vi "get wavefront.vi"(8 "error in":errorcluster, 11 "HasoSlopes in":refnum<class "HasoSlopes.lvclass">) -> (0 "error out":errorcluster, 1 "Pupil (new)":refnum<class "Pupil.lvclass">, 2 "Phase":refnum<class "Phase.lvclass">, 3 "HasoData out":refnum<class "HasoData.lvclass">, 5 "ComputePhaseSet.lvclass 2":refnum<class "ComputePhaseSet.lvclass">)   [LabVIEW 2020]
uses:
  Pupil.lvclass
  Phase.lvclass
  HasoSlopes.lvclass
  ComputePhaseSet.lvclass
  HasoData.lvclass
  WavefrontReconstructionMode.ctl
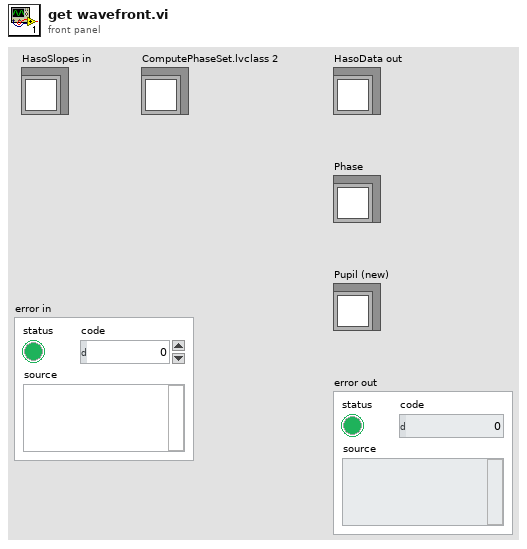
[diagram p1: front panel]
types:
  T1 = typedef "WavefrontReconstructionMode.ctl" = enum16{"None", "Modal_Legendre", "Modal_Zernike", "Zonal", "Modal_Zonal_Zernike", "Modal_Zonal_Legendre"}
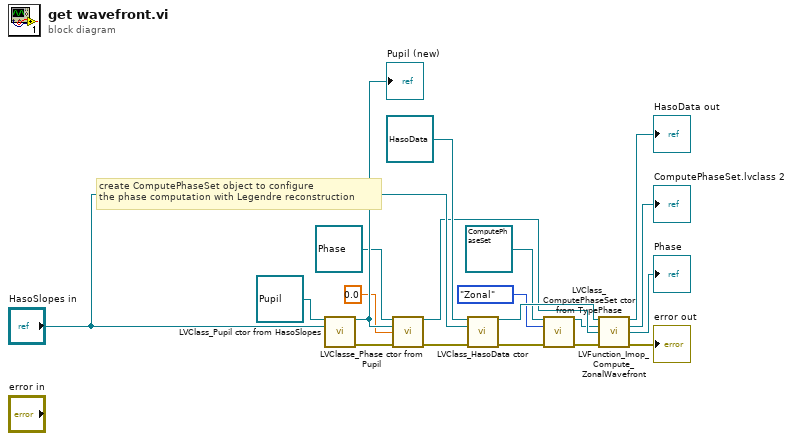
[diagram p0: block diagram]
diagram:
  # "create ComputePhaseSet object to configure\nthe phase computation with Legendre reconstruction"
  n1 = call "LVClass_Pupil ctor from HasoSlopes.vi"("Pupil (const)"=refnum<class "Pupil.lvclass"> refnum ("Pupil in"), "HasoSlopes"="HasoSlopes in") -> ("Pupil (new)"=w19:refnum<class "Pupil.lvclass">, "error out"=w6:errorcluster)  [unwired: 11 in, 1 out]
  "Pupil (new)" <- w19
  n2 = call "LVClasse_Phase ctor from Pupil.vi"("Phase (const)"=refnum<class "Phase.lvclass"> refnum ("Phase in"), "Pupil"=w19, "coef"=sgl 0.0, "error in (no error)"=w6) -> ("Phase (new)"=w8:refnum<class "Phase.lvclass">, "error out"=w12:errorcluster)  [unwired: 9 in, 1 out]
  n3 = call "LVClass_HasoData ctor.vi"("HasoData (const)"=refnum<class "HasoData.lvclass"> refnum ("HasoData in"), "HasoSlopes"="HasoSlopes in", "error in (no error)"=w12) -> ("HasoData (new)"=w16:refnum<class "HasoData.lvclass">, "error out"=w13:errorcluster)  [unwired: 10 in, 1 out]
  n4 = call "LVClass_ComputePhaseSet ctor from TypePhase.vi"("ComputePhaseSet (const)"=refnum<class "ComputePhaseSet.lvclass"> refnum ("ComputePhaseSet in"), "TypePhase"=WavefrontReconstructionMode."Zonal", "error in (no error)"=w13) -> ("ComputePhaseSet (new)"=w7:refnum<class "ComputePhaseSet.lvclass">, "error out"=w14:errorcluster)  [unwired: 11 in]
  n5 = call "LVFunction_Imop_Compute_ZonalWavefront.vi"("HasoData.lvclass"=w16, "ComputePhaseSet.lvclass"=w7, "Phase"=w8, "error constant"=w14) -> ("HasoData.lvclass (dup)"=→"HasoData out":refnum<class "HasoData.lvclass">, "ComputePhaseSet.lvclass 2"=→"ComputePhaseSet.lvclass 2":refnum<class "ComputePhaseSet.lvclass">, "Phase"=→"Phase":refnum<class "Phase.lvclass">, "error out"=→"error out":errorcluster)  [unwired: 8 in]
